vi "_init_assert_properties.vi"(8 "upstream error":errorcluster, 9 "Execution time (s)":dbl=-1.0, 10 "Asserted":bool, 11 "Assert in":refnum<class "Assert.lvclass">) -> (3 "Properties.Assert":refnum<class "Properties.Assert.lvclass">)   [LabVIEW 2013, in "Caraya.lvlib" / "Assert.lvclass"]
uses:
  Assert.lvclass
  Properties.Assert/Properties.Assert.lvclass
  Assert.lvclass/Assert.ctl
  Properties.Assert/Properties.Assert.lvclass/Properties.Assert.ctl
  Properties/Properties.lvclass
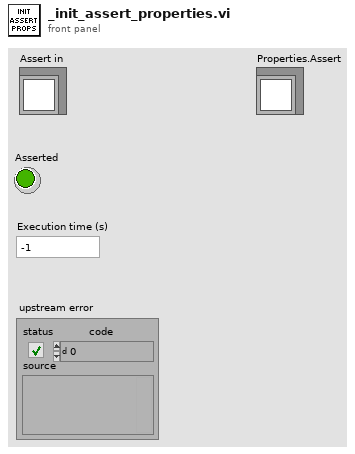
[diagram p1: front panel]
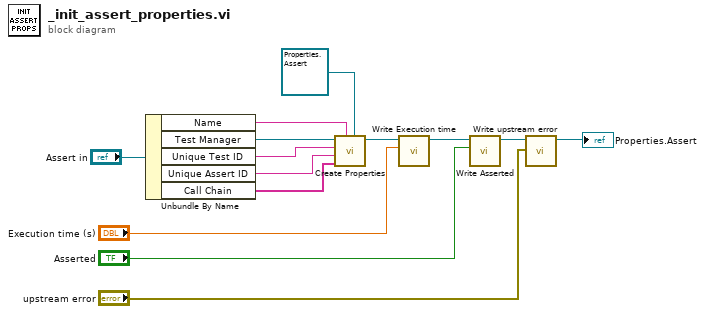
[diagram p0: block diagram]
diagram:
  n1 = Unbundle By Name("Assert in") -> ("Name"=w8:string, "Test Manager"=w12:refnum<class "Basic Test Manager.lvclass">, "Unique Test ID"=w11:string, "Unique Assert ID"=w10:string, "Call Chain"=w9:string[])
  n2 = call "Create Properties.vi"("Properties in"=refnum<class "Properties.Assert.lvclass"> refnum ("Caraya.lvlib:Properties.Assert.lvclass"), "label"=w8, "call-chain"=w9, "self-id"=w10, "owner-id"=w11, "Test Manager"=w12) -> ("Properties out"=w5:refnum<class "Properties.Assert.lvclass">)  [unwired: 5 in]
  n3 = call "Write Execution time.vi"("Execution time (s)"="Execution time (s)", "Properties.Assert in"=w5) -> ("Properties.Assert out"=w7:refnum<class "Properties.Assert.lvclass">)  [unwired: 9 in]
  n4 = call "Write Asserted.vi"("Asserted"="Asserted", "Properties.Assert in"=w7) -> ("Properties.Assert out"=w6:refnum<class "Properties.Assert.lvclass">)  [unwired: 9 in]
  n5 = call "Write upstream error.vi"("upstream-error"="upstream error", "Properties.Assert in"=w6) -> ("Properties.Assert out"=→"Properties.Assert":refnum<class "Properties.Assert.lvclass">)  [unwired: 9 in]
